vi "TEST_ConfigClass.vi"(8 "error in (no error)":errorcluster, 11 "ConfigClass in":refnum<class "ConfigClass.lvclass">) -> (0 "error out":errorcluster, 3 "ConfigClass out":refnum<class "ConfigClass.lvclass">)   [LabVIEW 2019, in "ConfigClass.lvlib" / "ConfigClass.lvclass"]
uses:
  ConfigClass.lvclass
panel:
  out "ok?":bool
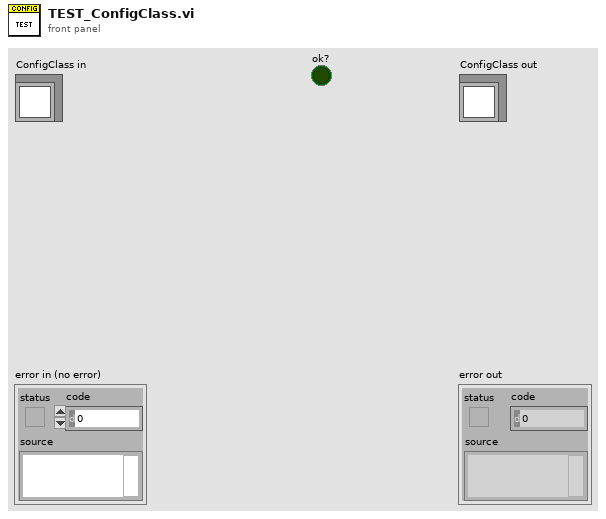
[diagram p1: front panel]
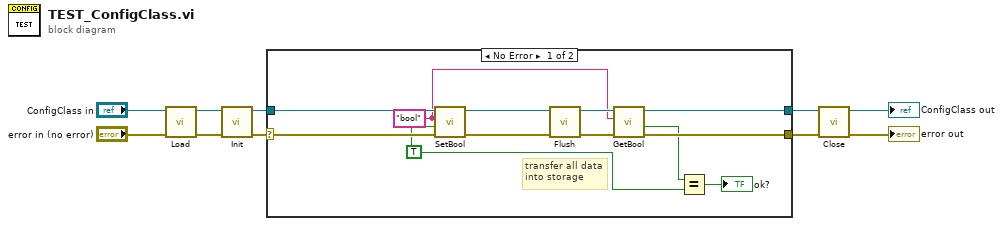
[diagram p0: block diagram]
diagram:
  n1 = call-dynamic "Load.vi"("error in (no error)"="error in (no error)", "ConfigClass_IN"="ConfigClass in") -> ("error out"=w5:errorcluster, "ConfigClass_OUT"=w6:refnum<class "ConfigClass.lvclass">)  [unwired: 8 in]
  n2 = call-dynamic "Init.vi"("error in (no error)"=w5, "ConfigClass_IN"=w6) -> ("error out"=w1:errorcluster, "ConfigClass_OUT"=w2:refnum<class "ConfigClass.lvclass">)  [unwired: 8 in]
  n3 = case shown="No Error" w1 {
    selector: w1 -> [w18 w24]
    tunnel: [w15 w24] -> w9
    tunnel: [w19 w23] -> w10
    tunnel: w2 -> [w21 w23]
    frame No Error {
      w12 = TRUE ("bool")
      w14 = "bool" ("key")
      # "transfer all data\ninto storage"
      n4 = call-dynamic "SetBool.vi"("error in (no error)"=w18, "bool"=w12, "key"=w14, "ConfigClass_IN"=w21) -> ("error out"=w17:errorcluster, "ConfigClass_OUT"=w20:refnum<class "ConfigClass.lvclass">)  [unwired: 6 in]
      n5 = call-dynamic "Flush.vi"("error in (no error)"=w17, "ConfigClass in"=w20) -> ("error out"=w16:errorcluster, "ConfigClass out"=w22:refnum<class "ConfigClass.lvclass">)  [unwired: 8 in]
      n6 = call-dynamic "GetBool.vi"("error in (no error)"=w16, "key"=w14, "ConfigClass_IN"=w22) -> ("error out"=w15:errorcluster, "bool"=w13:bool, "ConfigClass_OUT"=w19:refnum<class "ConfigClass.lvclass">)  [unwired: 6 in]
      n7 = Equal?(x=w13, y=w12) -> (x = y?=→"ok?":bool)
    }
    frame Error {
    }
  }
  n8 = call-dynamic "Close.vi"("error in (no error)"=w9, "ConfigClass_IN"=w10) -> ("error out"=→"error out":errorcluster, "ConfigClass_OUT"=→"ConfigClass out":refnum<class "ConfigClass.lvclass">)  [unwired: 8 in]
